vi "Ejemplo_FotoRamon.vi"() -> ()   [LabVIEW 2020]
uses:
  <vilib>/userdefined/High Color/IMAQdx.ctl
  <vilib>/vision/Image Controls.llb/IMAQ Image.ctl
  <vilib>/vision/driver/NI_Vision_Acquisition_Software.lvlib
  <vilib>/vision/NI_Vision_Development_Module.lvlib
panel:
  in  "Boolean":bool
  out "Captura":T1(plugin-control)
  in  "Stop Button":bool
  in  "Session In":T2
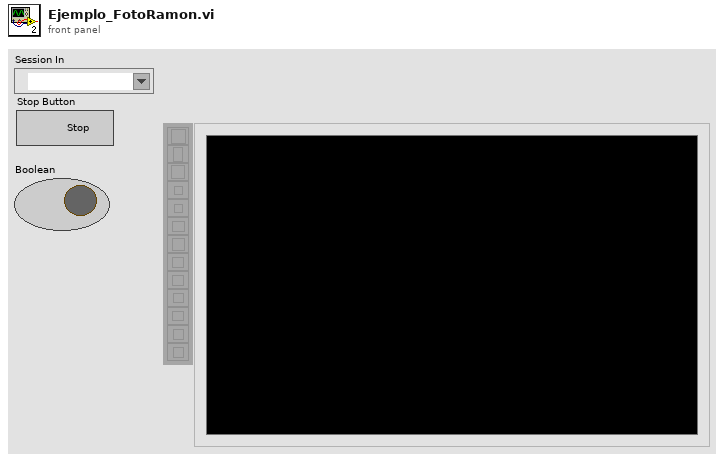
[diagram p1: front panel]
types:
  T1 = typedef "IMAQ Image.ctl" = refnum<image>
  T2 = typedef "IMAQdx.ctl" = refnum<k21>
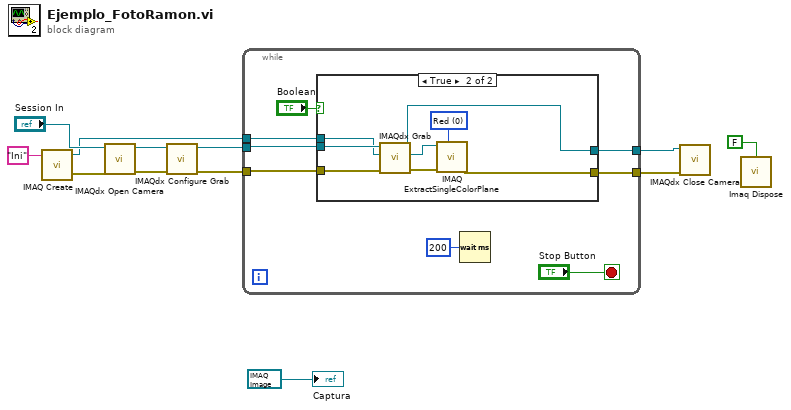
[diagram p0: block diagram]
diagram:
  n1 = call "IMAQ Create"("Image Name"="Ini") -> ("New Image"=w5:T1, "error out"=w11:errorcluster)  [unwired: 4 in]
  n2 = call <vilib>:"IMAQdx Open Camera.vi"("error in"=w11, "Session In"="Session In") -> ("error out"=w8:errorcluster, "Session Out"=w9:T2)  [unwired: 8 in]
  n3 = call <vilib>:"IMAQdx Configure Grab.vi"("error in"=w8, "Session In"=w9) -> ("error out"=w6:errorcluster, "Session Out"=w7:T2)  [unwired: 8 in]
  n4 = while {
    tunnel: w7 -> [w19]
    tunnel: w6 -> [w18]
    tunnel: w5 -> [w17]
    tunnel: [w16] -> w3
    tunnel: [w15] -> w2
    stop <- "Stop Button" stop-if-true
    n5 = case shown="True" "Boolean" {
      tunnel: w19 -> [w22 w27]
      tunnel: w18 -> [w21 w26]
      tunnel: w17 -> [_ w23]
      tunnel: [w21 w25] -> w16
      tunnel: [w22 w24] -> w15
      frame False {
      }
      frame True {
        w28 = 0 items=["Red", "Green", "Blue", "Hue", "Saturation", "Luminance", "Value", "Intensity"] ("Color Plane")
        n6 = call <vilib>:"IMAQdx Grab.vi"("error in"=w26, "Image In"=w23, "Session In"=w27) -> ("error out"=w29:errorcluster, "Image Out"=w30:T1, "Session Out"=w24:T2)  [unwired: 5 in, 1 out]
        n7 = call "IMAQ ExtractSingleColorPlane"("Color Plane"=w28, "error in (no error)"=w29, "Image Src"=w30) -> ("error out"=w25:errorcluster)  [unwired: 7 in, 1 out]
      }
    }
    n8 = Wait (ms)(milliseconds to wait=u32 200) -> ()  [unwired: 1 out]
  }
  n9 = call <vilib>:"IMAQdx Close Camera.vi"("error in"=w3, "Session In"=w2) -> ()  [unwired: 9 in, 1 out]
  n10 = call "Imaq Dispose"("All Images? (No)"=FALSE) -> ()  [unwired: 5 in, 1 out]
  "Captura" <- T1 refnum ("Captura")
